vi "Configure TTL Trigger.vi"(0 "VISA resource name":refnum<visa-resource-name>, 5 "TTL Trigger Mode (0:Trigger)":u16(ring) items=["Trigger", "Strobe"], 7 "Enable TTl Trigger (T: Enable)":bool=TRUE, 9 "TTL Trigger Source (0:BOT)":u16(ring) items=["Beginning of Transient Output (BOT)", "End of Transient Output (EOT)", "TTL Trigger List (LIST)"], 11 "error in (no error)":errorcluster) -> (4 "VISA resource name out":refnum<visa-resource-name>, 15 "error out":errorcluster)   [LabVIEW 2010, in "California Instruments iX Series.lvlib"]
doc: "Configures the TTL Trigger output located on the rear of the instrument. The output is part of the Auxiliary I/O Connector."
uses:
  <instrlib>/California Instruments iX Series/California Instruments iX Series.lvlib
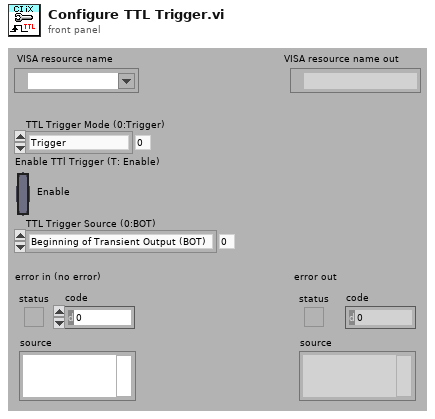
[diagram p1: front panel]
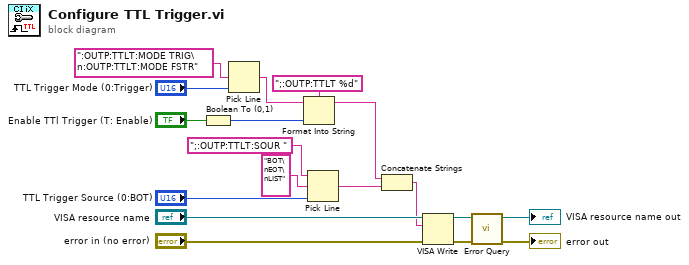
[diagram p0: block diagram]
diagram:
  n1 = Boolean To (0,1)(Boolean="Enable TTl Trigger (T: Enable)") -> (0, 1=w10:i16)
  n2 = Pick Line(multi-line string=":OUTP:TTLT:MODE TRIG\n:OUTP:TTLT:MODE FSTR", line index="TTL Trigger Mode (0:Trigger)") -> (output string=w7:string)  [unwired: 1 in]
  n3 = Format Into String(format string=";:OUTP:TTLT %d", initial string=w7, w10) -> (resulting string=w3:string)  [unwired: 1 in, 1 out]
  n4 = Pick Line(string ("")=";:OUTP:TTLT:SOUR ", multi-line string="BOT\nEOT\nLIST", line index="TTL Trigger Source (0:BOT)") -> (output string=w2:string)
  n5 = Concatenate Strings(w3, w2) -> (w1:string)
  n6 = VISA Write(VISA resource name="VISA resource name", write buffer=w1, error in (no error)="error in (no error)") -> (VISA resource name out=w16:refnum<visa-resource-name>, error out=w15:errorcluster)  [unwired: 1 out]
  n7 = call <instrlib>:"Error Query.vi"("error in (no error)"=w15, "VISA resource name"=w16) -> ("error out"=→"error out":errorcluster, "VISA resource name out"=→"VISA resource name out":refnum<visa-resource-name>)  [unwired: 6 in, 2 out]
